vi "HolatMecanums.vi"(5 "MaxOutput":dbl=500.0, 6 "AUTO TRACK BUTTON":bool, 7 "CAMERA X POS":dbl, 8 "ROBOT REVERSE":bool, 9 "STRAFE BUTTON":bool, 10 "Y AXIS":dbl, 11 "X AXIS":dbl) -> (0 "BackRight":dbl, 1 "BackLeft":dbl, 2 "FrontRight":dbl, 3 "FrontLeft":dbl)   [LabVIEW 2012]
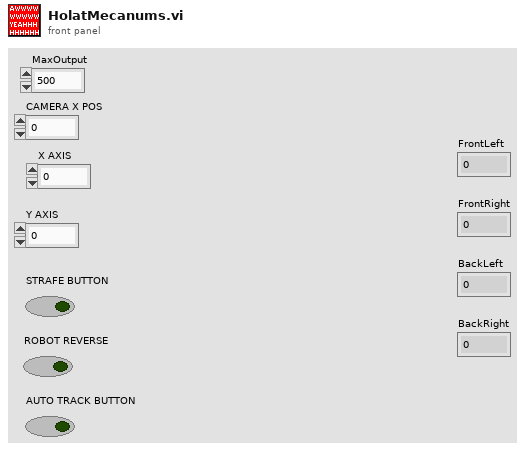
[diagram p1: front panel]
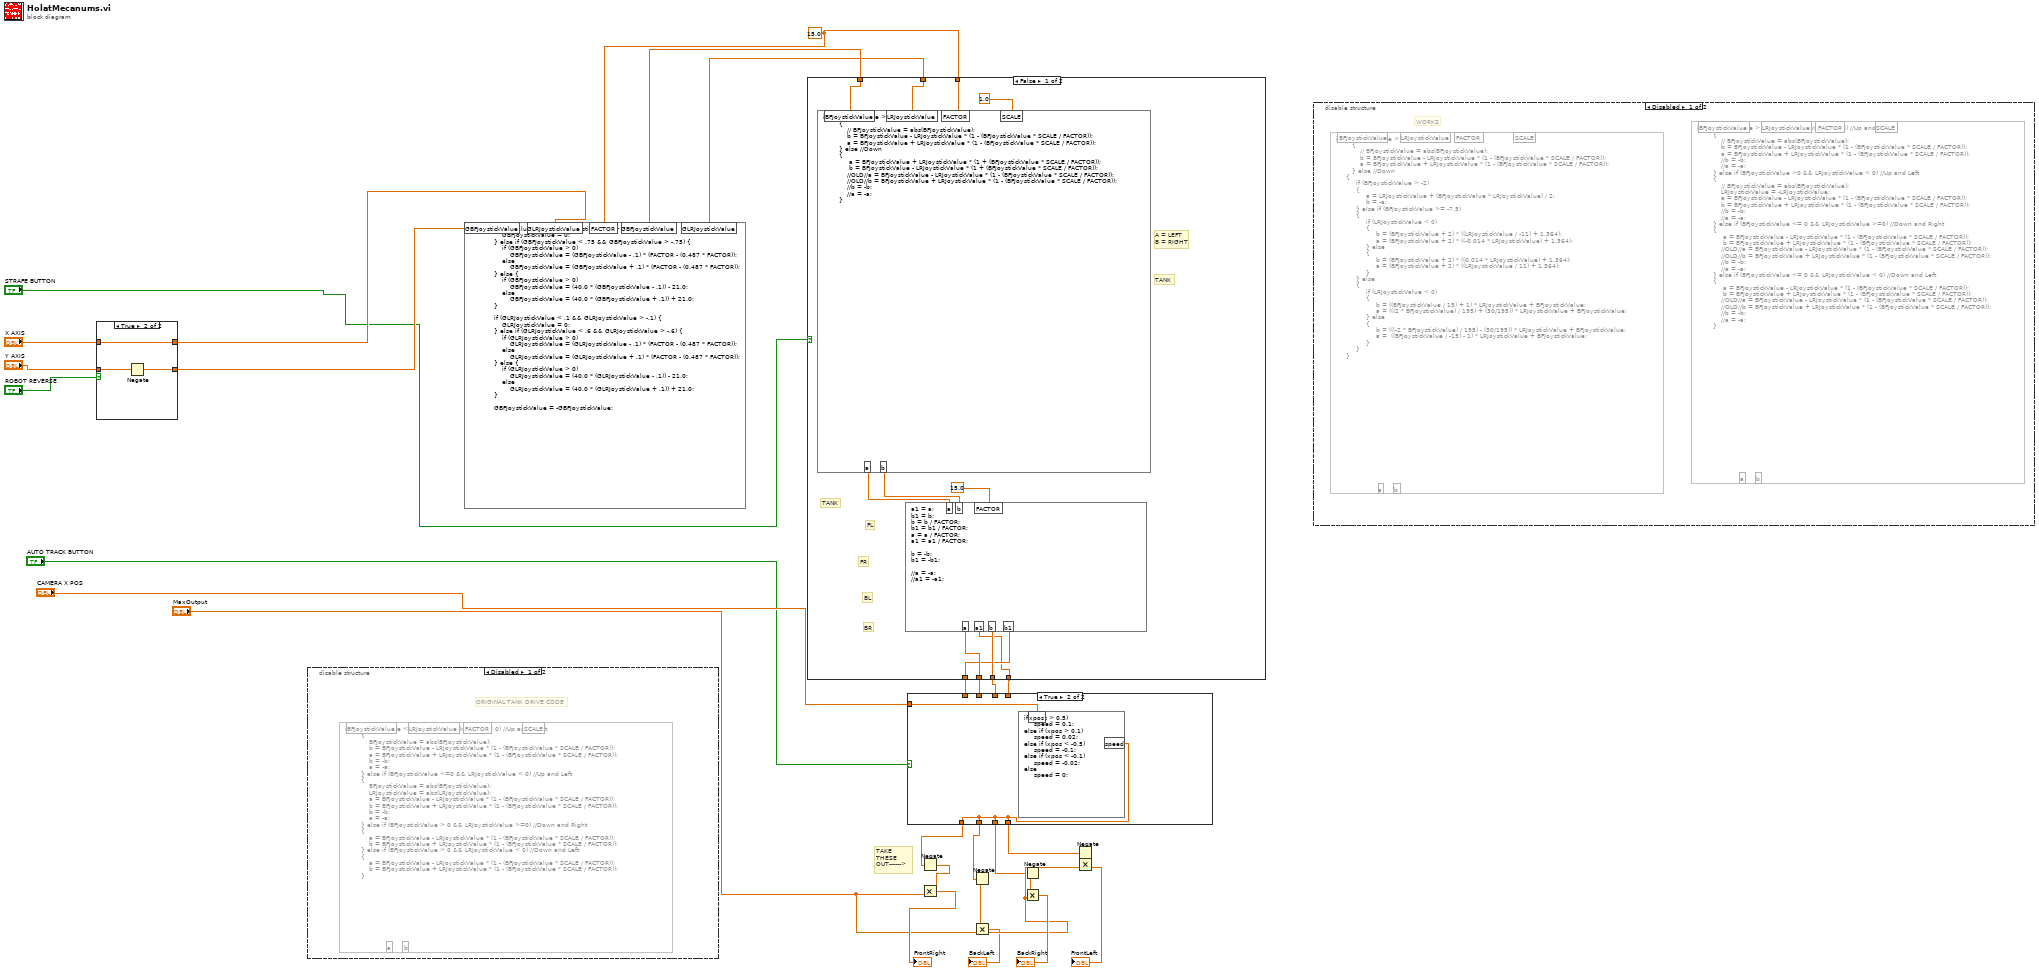
[diagram p0: block diagram]
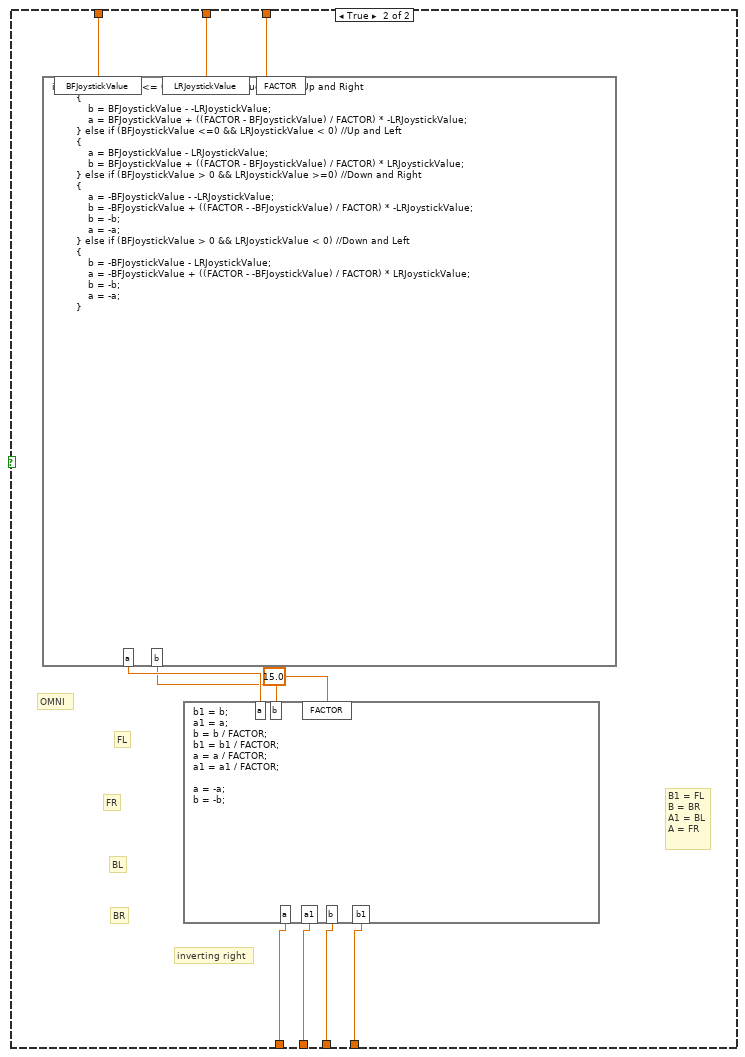
[diagram p6: hidden frame]
diagram:
  w28 = 15.0 ("input variable")
  # "TAKE\nTHESE\nOUT------>"
  n1 = case shown="True" "ROBOT REVERSE" {
    tunnel: [w30 w31] -> w25
    tunnel: [w29 w33] -> w24
    tunnel: "X AXIS" -> [w30 w31]
    tunnel: "Y AXIS" -> [w29 w32]
    frame False {
    }
    frame True {
      n2 = Negate(x=w32) -> (-x=w33:dbl)
    }
  }
  n3 = disable-structure shown="Disabled" {
    frame Disabled {
      # "ORIGINAL TANK DRIVE CODE"
      n4 = formula code="if (BFJoystickValue <= 0 && LRJoystickValue >= 0) //Up and Right\n        {\n            BFJoystickValue = abs(BFJoystickValue);\n            b = BFJoystickValue - LRJoystickValue * (1 - (BFJoystickValue * SCALE / FACTOR));\n            a = BFJoystickValue + LRJoystickValue * (1 - (BFJoystickValue * SCALE / FACTOR));\n            b = -b;\n            a = -a;\n        } else if (BFJoystickValue <=0 && LRJoystickValue < 0) //Up and Left\n        {\n            BFJoystickValue = abs(BFJoystickValue);\n            LRJoystickValue = abs(LRJoystickValue);\n            a = BFJoystickValue - LRJoystickValue * (1 - (BFJoystickValue * SCALE / FACTOR));\n            b = BFJoystickValue + LRJoystickValue * (1 - (BFJoystickValue * SCALE / FACTOR));\n            b = -b;\n            a = -a;\n        } else if (BFJoystickValue > 0 && LRJoystickValue >=0) //Down and Right\n        {\n            a = BFJoystickValue - LRJoystickValue * (1 - (BFJoystickValue * SCALE / FACTOR));\n            b = BFJoystickValue + LRJoystickValue * (1 - (BFJoystickValue * SCALE / FACTOR));\n        } else if (BFJoystickValue > 0 && LRJoystickValue < 0) //Down and Left\n        {\n            a = BFJoystickValue - LRJoystickValue * (1 - (BFJoystickValue * SCALE / FACTOR));\n            b = BFJoystickValue + LRJoystickValue * (1 - (BFJoystickValue * SCALE / FACTOR));\n        }"() -> ()  [unwired: 4 in, 2 out]
    }
    frame Enabled {
    }
  }
  n5 = formula code="if (GBFJoystickValue < .1 && GBFJoystickValue > -.1) {\n                GBFJoystickValue = 0;\n            } else if (GBFJoystickValue < .75 && GBFJoystickValue > -.75) {\n                if (GBFJoystickValue > 0)\n                    GBFJoystickValue = (GBFJoystickValue - .1) * (FACTOR - (0.487 * FACTOR));\n                else\n                    GBFJoystickValue = (GBFJoystickValue + .1) * (FACTOR - (0.487 * FACTOR));\n            } else {\n                if (GBFJoystickValue > 0)\n                    GBFJoystickValue = (40.0 * (GBFJoystickValue - .1)) - 21.0;\n                else\n                    GBFJoystickValue = (40.0 * (GBFJoystickValue + .1)) + 21.0;\n            }\n\n            if (GLRJoystickValue < .1 && GLRJoystickValue > -.1) {\n                GLRJoystickValue = 0;\n            } else if (GLRJoystickValue < .6 && GLRJoystickValue > -.6) {\n                if (GLRJoystickValue > 0)\n                    GLRJoystickValue = (GLRJoystickValue - .1) * (FACTOR - (0.487 * FACTOR));\n                else\n                    GLRJoystickValue = (GLRJoystickValue + .1) * (FACTOR - (0.487 * FACTOR));\n            } else {\n                if (GLRJoystickValue > 0)\n                    GLRJoystickValue = (40.0 * (GLRJoystickValue - .1)) - 21.0;\n                else\n                    GLRJoystickValue = (40.0 * (GLRJoystickValue + .1)) + 21.0;\n            }\n\n            GBFJoystickValue = -GBFJoystickValue;"("FACTOR"=w28, "GBFJoystickValue"=w24, "GLRJoystickValue"=w25) -> ("GBFJoystickValue"=w27:dbl, "GLRJoystickValue"=w26:dbl)
  n6 = case shown="False" "STRAFE BUTTON" {
    tunnel: w28 -> [w39 w51]
    tunnel: [w40 w50] -> w3
    tunnel: [w41 w47] -> w9
    tunnel: [w43 w49] -> w6
    tunnel: [w42 w48] -> w8
    tunnel: w27 -> [w36 w46]
    tunnel: w26 -> [w37 w45]
    frame False {
      # "A = LEFT\nB = RIGHT"
      # "BR"
      # "BL"
      # "FR"
      # "FL"
      # "TANK"
      # "TANK"
      n7 = formula code="if (BFJoystickValue > 0) //Up\n        {\n            // BFJoystickValue = abs(BFJoystickValue);\n            b = BFJoystickValue - LRJoystickValue * (1 - (BFJoystickValue * SCALE / FACTOR));\n            a = BFJoystickValue + LRJoystickValue * (1 - (BFJoystickValue * SCALE / FACTOR));\n        } else //Down\n        {\n             a = BFJoystickValue + LRJoystickValue * (1 + (BFJoystickValue * SCALE / FACTOR));\n             b = BFJoystickValue - LRJoystickValue * (1 + (BFJoystickValue * SCALE / FACTOR));\n            //OLD//a = BFJoystickValue - LRJoystickValue * (1 - (BFJoystickValue * SCALE / FACTOR));\n            //OLD//b = BFJoystickValue + LRJoystickValue * (1 - (BFJoystickValue * SCALE / FACTOR));\n            //b = -b;\n            //a = -a;\n        }"("BFJoystickValue"=w36, "LRJoystickValue"=w37, "FACTOR"=w39, "SCALE"=1.0 ("input variable")) -> ("a"=w34:dbl, "b"=w35:dbl)
      n8 = formula code="a1 = a;\nb1 = b;\nb = b / FACTOR;\nb1 = b1 / FACTOR;\na = a / FACTOR;\na1 = a1 / FACTOR;\n\nb = -b;\nb1 = -b1;\n\n//a = -a;\n//a1 = -a1;"("a"=w34, "b"=w35, "FACTOR"=15.0 ("input variable")) -> ("a"=w42:dbl, "a1"=w40:dbl, "b"=w43:dbl, "b1"=w41:dbl)
    }
    frame True {
      # "inverting right"
      # "B1 = FL\nB = BR\nA1 = BL\nA = FR"
      # "BR"
      # "BL"
      # "FR"
      # "FL"
      # "OMNI"
      n9 = formula code="if (BFJoystickValue <= 0 && LRJoystickValue >= 0) //Up and Right\n        {\n            b = BFJoystickValue - -LRJoystickValue;\n            a = BFJoystickValue + ((FACTOR - BFJoystickValue) / FACTOR) * -LRJoystickValue;\n        } else if (BFJoystickValue <=0 && LRJoystickValue < 0) //Up and Left\n        {\n            a = BFJoystickValue - LRJoystickValue;\n            b = BFJoystickValue + ((FACTOR - BFJoystickValue) / FACTOR) * LRJoystickValue;\n        } else if (BFJoystickValue > 0 && LRJoystickValue >=0) //Down and Right\n        {\n            a = -BFJoystickValue - -LRJoystickValue;\n            b = -BFJoystickValue + ((FACTOR - -BFJoystickValue) / FACTOR) * -LRJoystickValue;\n            b = -b;\n            a = -a;\n        } else if (BFJoystickValue > 0 && LRJoystickValue < 0) //Down and Left\n        {\n            b = -BFJoystickValue - LRJoystickValue;\n            a = -BFJoystickValue + ((FACTOR - -BFJoystickValue) / FACTOR) * LRJoystickValue;\n            b = -b;\n            a = -a;\n        }"("BFJoystickValue"=w46, "LRJoystickValue"=w45, "FACTOR"=w51) -> ("a"=w54:dbl, "b"=w53:dbl)
      n10 = formula code="b1 = b;\na1 = a;\nb = b / FACTOR;\nb1 = b1 / FACTOR;\na = a / FACTOR;\na1 = a1 / FACTOR;\n\na = -a;\nb = -b;"("a"=w54, "b"=w53, "FACTOR"=15.0 ("input variable")) -> ("a"=w47:dbl, "a1"=w48:dbl, "b"=w49:dbl, "b1"=w50:dbl)
    }
  }
  n11 = case shown="True" "AUTO TRACK BUTTON" {
    tunnel: [w58 w59] -> w10
    tunnel: w9 -> [w58 _]
    tunnel: w8 -> [w57 _]
    tunnel: [w57 w59] -> w7
    tunnel: w6 -> [w56 _]
    tunnel: [w56 w59] -> w5
    tunnel: [w55 w59] -> w4
    tunnel: w3 -> [w55 _]
    tunnel: "CAMERA X POS" -> [_ w60]
    frame False {
    }
    frame True {
      n12 = formula code="if (xpos > 0.5)\n     speed = 0.1;\nelse if (xpos > 0.1)\n     speed = 0.02;\nelse if (xpos < -0.5)\n     speed = -0.1;\nelse if (xpos < -0.1)\n     speed = -0.02;\nelse \n     speed = 0;"("xpos"=w60) -> ("speed"=w59:dbl)
    }
  }
  n13 = Negate(x=w10) -> (-x=w16:dbl)
  n14 = Multiply(x=w16, y="MaxOutput") -> (x*y=→"FrontRight":dbl)
  n15 = Negate(x=w7) -> (-x=w15:dbl)
  n16 = Multiply(x=w15, y="MaxOutput") -> (x*y=→"BackLeft":dbl)
  n17 = Negate(x=w5) -> (-x=w14:dbl)
  n18 = Multiply(x=w14, y="MaxOutput") -> (x*y=→"BackRight":dbl)
  n19 = Negate(x=w4) -> (-x=w13:dbl)
  n20 = Multiply(x=w13, y="MaxOutput") -> (x*y=→"FrontLeft":dbl)
  n21 = disable-structure shown="Disabled" {
    frame Disabled {
      # "WORKS"
      n22 = formula code="if (BFJoystickValue > 0) //Up\n        {\n            // BFJoystickValue = abs(BFJoystickValue);\n            b = BFJoystickValue - LRJoystickValue * (1 - (BFJoystickValue * SCALE / FACTOR));\n            a = BFJoystickValue + LRJoystickValue * (1 - (BFJoystickValue * SCALE / FACTOR));\n        } else //Down\n     {\n          if (BFJoystickValue > -2)\n          {\n               a = LRJoystickValue + (BFJoystickValue * LRJoystickValue) / 2;\n               b = -a;\n          } else if (BFJoystickValue >= -7.5)\n          {\n               if (LRJoystickValue < 0)\n               {\n                    b = (BFJoystickValue + 2) * ((LRJoystickValue / -11) + 1.364);\n                    a = (BFJoystickValue + 2) * ((-0.014 * LRJoystickValue) + 1.364);\n               } else\n               {\n                    b = (BFJoystickValue + 2) * ((0.014 * LRJoystickValue) + 1.364);\n                    a = (BFJoystickValue + 2) * ((LRJoystickValue / 11) + 1.364);\n               }\n          } else\n          {\n               if (LRJoystickValue < 0)\n               {\n                    b = ((BFJoystickValue / 15) + 1) * LRJoystickValue + BFJoystickValue;\n                    a = (((2 * BFJoystickValue) / 195) + (30/195)) * LRJoystickValue + BFJoystickValue;\n               } else\n               {\n                    b = (((-2 * BFJoystickValue) / 195) - (30/195)) * LRJoystickValue + BFJoystickValue;\n                    a =  ((BFJoystickValue / -15) - 1) * LRJoystickValue + BFJoystickValue;\n               }\n          }\n     }"() -> ()  [unwired: 4 in, 2 out]
      n23 = formula code="if (BFJoystickValue > 0 && LRJoystickValue >= 0) //Up and Right\n        {\n            // BFJoystickValue = abs(BFJoystickValue);\n            b = BFJoystickValue - LRJoystickValue * (1 - (BFJoystickValue * SCALE / FACTOR));\n            a = BFJoystickValue + LRJoystickValue * (1 - (BFJoystickValue * SCALE / FACTOR));\n            //b = -b;\n            //a = -a;\n        } else if (BFJoystickValue >0 && LRJoystickValue < 0) //Up and Left\n        {\n            // BFJoystickValue = abs(BFJoystickValue);\n            LRJoystickValue = -LRJoystickValue;\n            a = BFJoystickValue - LRJoystickValue * (1 - (BFJoystickValue * SCALE / FACTOR));\n            b = BFJoystickValue + LRJoystickValue * (1 - (BFJoystickValue * SCALE / FACTOR));\n            //b = -b;\n            //a = -a;\n        } else if (BFJoystickValue <= 0 && LRJoystickValue >=0) //Down and Right\n        {\n             a = BFJoystickValue - LRJoystickValue * (1 - (BFJoystickValue * SCALE / FACTOR));\n             b = BFJoystickValue + LRJoystickValue * (1 - (BFJoystickValue * SCALE / FACTOR));\n            //OLD//a = BFJoystickValue - LRJoystickValue * (1 - (BFJoystickValue * SCALE / FACTOR));\n            //OLD//b = BFJoystickValue + LRJoystickValue * (1 - (BFJoystickValue * SCALE / FACTOR));\n            //b = -b;\n            //a = -a;\n        } else if (BFJoystickValue <= 0 && LRJoystickValue < 0) //Down and Left\n        {\n             a = BFJoystickValue - LRJoystickValue * (1 - (BFJoystickValue * SCALE / FACTOR));\n             b = BFJoystickValue + LRJoystickValue * (1 - (BFJoystickValue * SCALE / FACTOR));\n            //OLD//a = BFJoystickValue - LRJoystickValue * (1 - (BFJoystickValue * SCALE / FACTOR));\n            //OLD//b = BFJoystickValue + LRJoystickValue * (1 - (BFJoystickValue * SCALE / FACTOR));\n            //b = -b;\n            //a = -a;\n        }"() -> ()  [unwired: 4 in, 2 out]
    }
    frame Enabled {
    }
  }
